vi "Mag Volt Sweep.vi"() -> ()   [LabVIEW 2012]
uses:
  <vilib>/Utility/file.llb/Write To Spreadsheet File (DBL).vi
panel:
  in  "file path (dialog if empty)":path
  in  "Numeric":i32
  in  "Channel":u16
  out "XY Graph 3":cluster{"Y":dbl[], "Y":dbl[]}[](graph)
  out "XY Graph 2":cluster{"Y":dbl[], "Y":dbl[]}[](graph)
  out "XY Graph":cluster{"Y":dbl[], "Y":dbl[]}[](graph)
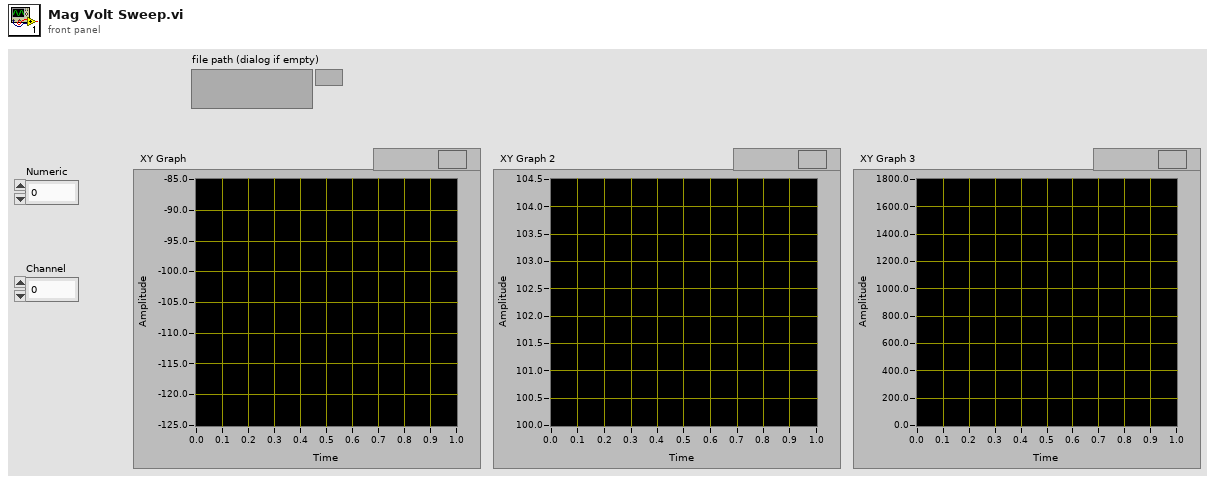
[diagram p1: front panel]
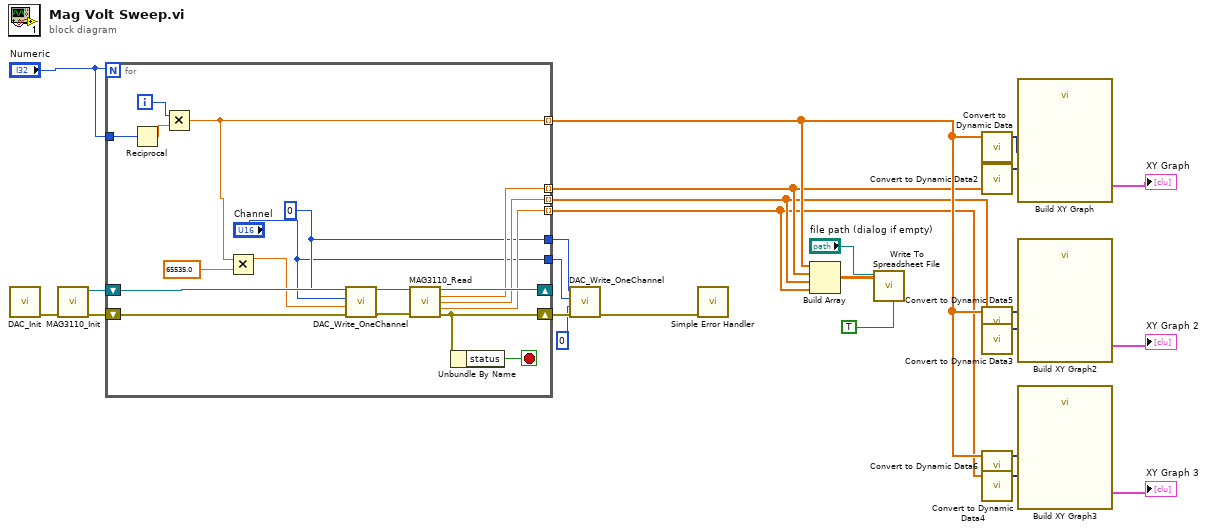
[diagram p0: block diagram]
diagram:
  n1 = call "DAC_Init.vi"() -> ("error out"=w25:errorcluster)  [unwired: 11 in]
  n2 = call "MAG3110_Init.vi"("error in (no error)"=w25) -> ("VISA resource name out"=w24:refnum<visa-resource-name>, "error out"=w23:errorcluster)  [unwired: 8 in]
  n3 = for {
    N: "Numeric" -> [_]
    shift-right: [w41] -> _
    shift-left: w24 -> [w42]
    shift-right: [w32] -> w12
    shift-left: w23 -> [w35]
    tunnel: "Numeric" -> [w40]
    tunnel: [w31] -> w7 mode=indexing
    tunnel: [w30] -> w6 mode=indexing
    tunnel: [w29] -> w5 mode=indexing
    tunnel: [w28] -> w4 mode=indexing
    tunnel: [w27] -> w11
    tunnel: ["Channel"] -> w10
    i -> [w39]
    stop <- w33 stop-if-true
    w27 = u64 0 ("DeviceIndex")
    n4 = Reciprocal(x=w40) -> (1/x=w38:dbl)
    n5 = Multiply(x=w39, y=w38) -> (x*y=w31:dbl)
    n6 = Multiply(x=w31, y=65535.0) -> (x*y=w36:dbl)
    n7 = call "DAC_Write_OneChannel.vi"("error in (no error)"=w35, "Value"=w36, "Channel"="Channel", "DeviceIndex"=w27) -> ("error out"=w34:errorcluster)  [unwired: 6 in, 1 out]
    n8 = call "MAG3110_Read.vi"("VISA resource name"=w42, "error in (no error)"=w34) -> ("VISA resource name out"=w41:refnum<visa-resource-name>, "X (uT)"=w30:dbl, "Y (uT)"=w29:dbl, "Z (uT)"=w28:dbl, "error out"=w32:errorcluster)  [unwired: 9 in]
    n9 = Unbundle By Name(w32) -> ("status"=w33:bool)
  }
  n10 = call "DAC_Write_OneChannel.vi"("error in (no error)"=w12, "Value"=u16 0, "Channel"=w10, "DeviceIndex"=w11) -> ("error out"=w8:errorcluster)  [unwired: 6 in, 1 out]
  n11 = call <vilib>:"Simple Error Handler.vi"("error in (no error)"=w8) -> ()  [unwired: 4 in, 5 out]
  n12 = Build Array(w7, w6, w5, w4) -> (w3:dbl[][])
  n13 = call-poly <vilib>:"Write To Spreadsheet File.vi"("transpose? (no:F)"=TRUE, "2D data"=w3, "file path (dialog if empty)"="file path (dialog if empty)") -> ()  [unwired: 5 in, 1 out]
  n14 = call "Convert to Dynamic Data"("Array"=w7) -> ("Dynamic Data Type"=w20:dynamicdata)  [unwired: 3 in]
  n15 = call "Convert to Dynamic Data2"("Array"=w6) -> ("Dynamic Data Type"=w19:dynamicdata)  [unwired: 3 in]
  n16 = call "Convert to Dynamic Data5"("Array"=w7) -> ("Dynamic Data Type"=w16:dynamicdata)  [unwired: 3 in]
  n17 = call "Convert to Dynamic Data3"("Array"=w5) -> ("Dynamic Data Type"=w18:dynamicdata)  [unwired: 3 in]
  n18 = call "Convert to Dynamic Data6"("Array"=w7) -> ("Dynamic Data Type"=w15:dynamicdata)  [unwired: 3 in]
  n19 = call "Convert to Dynamic Data4"("Array"=w4) -> ("Dynamic Data Type"=w17:dynamicdata)  [unwired: 3 in]
  n20 = call "Build XY Graph"("Y Input"=w19, "X Input"=w20) -> ("XY Graph"=→"XY Graph":cluster{"Y":dbl[], "Y":dbl[]}[])  [unwired: 3 in, 6 out]
  n21 = call "Build XY Graph2"("Y Input"=w18, "X Input"=w16) -> ("XY Graph"=→"XY Graph 2":cluster{"Y":dbl[], "Y":dbl[]}[])  [unwired: 3 in, 6 out]
  n22 = call "Build XY Graph3"("Y Input"=w17, "X Input"=w15) -> ("XY Graph"=→"XY Graph 3":cluster{"Y":dbl[], "Y":dbl[]}[])  [unwired: 3 in, 6 out]
